vi "FT_Read_FT232H_EEPROM.vi"(0 "Handle":u32) -> (1 "FT_Status":u32(ring) items=["FT_OK", "FT_INVALID_HANDLE", "FT_DEVICE_NOT_FOUND", "FT_DEVICE_NOT_OPENED", "FT_IO_ERROR", "FT_INSUFFICIENT_RESOURCES", "FT_INVALID_PARAMETER", "FT_INVALID_BAUD_RATE", "FT_DEVICE_NOT_OPENED_FOR_ERASE", "FT_DEVICE_NOT_OPENED_FOR_WRITE", "FT_FAILED_TO_WRITE_DEVICE", "FT_EEPROM_READ_FAILED", "FT_EEPROM_WRITE_FAILED", "FT_EEPROM_ERASE_FAILED", "FT_EEPROM_NOT_PRESENT", "FT_EEPROM_NOT_PROGRAMMED", "FT_INVALID_ARGS", "FT_NOT_SUPPORTED", "FT_OTHER_ERROR"], 2 "FT232H EEPROM Contents":T1={"Vendor ID"=0, "Product ID"=0, "Manufacturer"="", "Manufacturer ID"="", "Description"="", "Serial Number"="", "Max Power (mA)"=0, "PnP"=0, "Self Powered"=0, "Remote Wake-Up"=0, "Pull Down Enable"=0, "Serial Number Enable"=0, "AC Slow Slew"=0, "AC Schmitt Input"=0, "AC Drive Current"=4, "AD Slow Slew"=0, "AD Schmitt Input"=0, "AD Drive Current"=4, "CBus0"=0, "CBus1"=0, "CBus2"=0, "CBus3"=0, "CBus4"=0, "CBus5"=0, "CBus6"=0, "CBus7"=0, "CBus8"=0, "CBus9"=0, "Is 245 FIFO"=0, "Is CPU FIFO"=0, "Is Fast Serial"=0, "Is FT1248"=0, "FT1248 Clock Polarity"=0, "FT1248 Bit Order"=0, "FT1248 Flow Control"=0, "Is VCP"=0, "Power Save"=0} {"Power Save" items=["Disabled", "Enabled"]; "Is VCP" items=["D2XX", "VCP"]; "FT1248 Flow Control" items=["Disabled", "Enabled"]; "FT1248 Bit Order" items=["MSB", "LSB"]; "FT1248 Clock Polarity" items=["Idle Low", "Idle High"]; "Is FT1248" items=["Disabled", "Enabled"]; "Is Fast Serial" items=["Disabled", "Enabled"]; "Is CPU FIFO" items=["Disabled", "Enabled"]; "Is 245 FIFO" items=["UART", "FIFO"]; "CBus9" items=["TRISTATE", "RXLED#", "TXLED#", "TX & RXLED#", "PWREN#", "SLEEP#", "DRIVE 0", "DRIVE 1", "IO Mode", "TXDEN#", "30MHz Clock", "15MHz Clock", "7.5MHz Clock"]; "CBus8" items=["TRISTATE", "RXLED#", "TXLED#", "TX & RXLED#", "PWREN#", "SLEEP#", "DRIVE 0", "DRIVE 1", "IO Mode", "TXDEN#", "30MHz Clock", "15MHz Clock", "7.5MHz Clock"]; "CBus7" items=["TRISTATE", "RXLED#", "TXLED#", "TX & RXLED#", "PWREN#", "SLEEP#", "DRIVE 0", "DRIVE 1", "IO Mode", "TXDEN#", "30MHz Clock", "15MHz Clock", "7.5MHz Clock"]; "CBus6" items=["TRISTATE", "RXLED#", "TXLED#", "TX & RXLED#", "PWREN#", "SLEEP#", "DRIVE 0", "DRIVE 1", "IO Mode", "TXDEN#", "30MHz Clock", "15MHz Clock", "7.5MHz Clock"]; "CBus5" items=["TRISTATE", "RXLED#", "TXLED#", "TX & RXLED#", "PWREN#", "SLEEP#", "DRIVE 0", "DRIVE 1", "IO Mode", "TXDEN#", "30MHz Clock", "15MHz Clock", "7.5MHz Clock"]; "CBus4" items=["TRISTATE", "RXLED#", "TXLED#", "TX & RXLED#", "PWREN#", "SLEEP#", "DRIVE 0", "DRIVE 1", "IO Mode", "TXDEN#", "30MHz Clock", "15MHz Clock", "7.5MHz Clock"]; "CBus3" items=["TRISTATE", "RXLED#", "TXLED#", "TX & RXLED#", "PWREN#", "SLEEP#", "DRIVE 0", "DRIVE 1", "IO Mode", "TXDEN#", "30MHz Clock", "15MHz Clock", "7.5MHz Clock"]; "CBus2" items=["TRISTATE", "RXLED#", "TXLED#", "TX & RXLED#", "PWREN#", "SLEEP#", "DRIVE 0", "DRIVE 1", "IO Mode", "TXDEN#", "30MHz Clock", "15MHz Clock", "7.5MHz Clock"]; "CBus1" items=["TRISTATE", "RXLED#", "TXLED#", "TX & RXLED#", "PWREN#", "SLEEP#", "DRIVE 0", "DRIVE 1", "IO Mode", "TXDEN#", "30MHz Clock", "15MHz Clock", "7.5MHz Clock"]; "CBus0" items=["TRISTATE", "RXLED#", "TXLED#", "TX & RXLED#", "PWREN#", "SLEEP#", "DRIVE 0", "DRIVE 1", "IO Mode", "TXDEN#", "30MHz Clock", "15MHz Clock", "7.5MHz Clock"]; "AD Drive Current" items=["4mA"=4, "8mA"=8, "12mA"=12, "16mA"=16]; "AD Schmitt Input" items=["Disabled", "Enabled"]; "AD Slow Slew" items=["Disabled", "Enabled"]; "AC Drive Current" items=["4mA"=4, "8mA"=8, "12mA"=12, "16mA"=16]; "AC Schmitt Input" items=["Disabled", "Enabled"]; "AC Slow Slew" items=["Disabled", "Enabled"]; "Serial Number Enable" items=["Disabled", "Enabled"]; "Pull Down Enable" items=["Disabled", "Enabled"]; "Remote Wake-Up" items=["Disabled", "Enabled"]; "Self Powered" items=["Bus Powered", "Self Powered"]; "PnP" items=["Disabled", "Enabled"]; "Product ID" format="%x"; "Vendor ID" format="%x"})   [LabVIEW 2020]
uses:
  GEA3 DLL Source/ftd2xx.dll
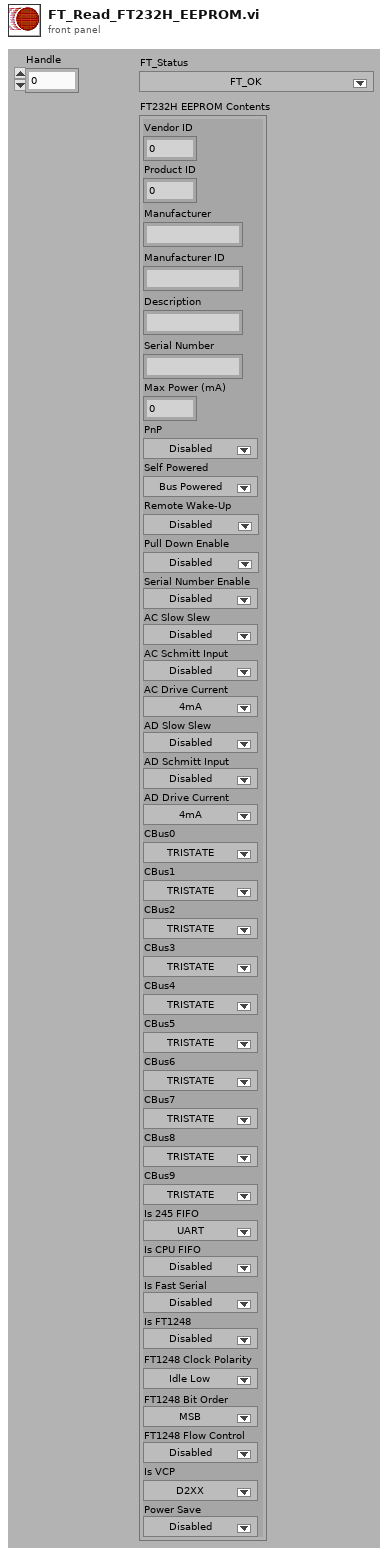
[diagram p1: front panel]
types:
  T1 = cluster{"Vendor ID":u16, "Product ID":u16, "Manufacturer":string, "Manufacturer ID":string, "Description":string, "Serial Number":string, "Max Power (mA)":u16, "PnP":u16, "Self Powered":u16, "Remote Wake-Up":u16, "Pull Down Enable":u8, "Serial Number Enable":u8, "AC Slow Slew":u8, "AC Schmitt Input":u8, "AC Drive Current":u8, "AD Slow Slew":u8, "AD Schmitt Input":u8, "AD Drive Current":u8, "CBus0":u8, "CBus1":u8, "CBus2":u8, "CBus3":u8, "CBus4":u8, "CBus5":u8, "CBus6":u8, "CBus7":u8, "CBus8":u8, "CBus9":u8, "Is 245 FIFO":u8, "Is CPU FIFO":u8, "Is Fast Serial":u8, "Is FT1248":u8, "FT1248 Clock Polarity":u8, "FT1248 Bit Order":u8, "FT1248 Flow Control":u8, "Is VCP":u8, "Power Save":u8}
  T2 = cluster{"Signature 1":u32, "Signature 2":u32, "Version":u32, "Vendor ID":u16, "Product ID":u16, "Manufacturer":u32, "Manufacturer ID":u32, "Description":u32, "Serial Number":u32, "Max Power (mA)":u16, "PnP":u16, "Self Powered":u16, "Remote Wake-Up":u16, "Rev4":u8, "Iso In":u8, "Iso Out":u8, "Pull Down Enable":u8, "Serial Number Enable":u8, "USB Version Enable":u8, "USB Version":u16, "Rev5":u8, "Iso In A":u8, "Iso In B":u8, "Iso Out A":u8, "Iso Out B":u8, "Pull Down Enable 5":u8, "Serial Number Enable 5":u8, "USB Version Enable 5":u8, "USB Version 5":u16, "A Is High Current":u8, "B Is High Current":u8, "A Is 245 FIFO":u8, "A Is CPU FIFO":u8, "A Is Fast Serial":u8, "A Is VCP":u8, "B Is 245 FIFO":u8, "B Is CPU FIFO":u8, "B Is Fast Serial":u8, "B Is VCP":u8, "Use Ext Osc":u8, "High Drive IOs":u8, "Endpoint Size":u8, "Pull Down Enable R":u8, "Serial Number Enable R":u8, "Invert TXD":u8, "Invert RXD":u8, "Invert RTS":u8, "Invert CTS":u8, "Invert DTR":u8, "Invert DSR":u8, "Invert DCD":u8, "Invert RI":u8, "CBus0":u8, "CBus1":u8, "CBus2":u8, "CBus3":u8, "CBus4":u8, "R Is VCP":u8, "Pull Down Enable 7":u8, "Serial Number Enable 7":u8, "AL Slow Slew":u8, "AL Schmitt Input":u8, "AL Drive Current":u8, "AH Slow Slew":u8, "AH Schmitt Input":u8, "AH Drive Current":u8, "BL Slow Slew":u8, "BL Schmitt Input":u8, "BL Drive Current":u8, "BH Slow Slew":u8, "BH Schmitt Input":u8, "BH Drive Current":u8, "A Is 245 FIFO 7":u8, "A Is CPU FIFO 7":u8, "A Is Fast Serial 7":u8, "A Is VCP 7":u8, "B Is 245 FIFO 7":u8, "B Is CPU FIFO 7":u8, "B Is Fast Serial 7":u8, "B Is VCP 7":u8, "PowerSaveEnable":u8, "Pull Down Enable 8":u8, "Serial Number Enable 8":u8, "A Slow Slew":u8, "A Schmitt Input":u8, "A Drive Current":u8, "B Slow Slew":u8, "B Schmitt Input":u8, "B Drive Current":u8, "C Slow Slew":u8, "C Schmitt Input":u8, "C Drive Current":u8, "D Slow Slew":u8, "D Schmitt Input":u8, "D Drive Current":u8, "A RI Is TXDEN":u8, "B RI Is TXDEN":u8, "C RI Is TXDEN":u8, "D RI Is TXDEN":u8, "A Is VCP 8":u8, "B Is VCP 8":u8, "C Is VCP 8":u8, "D Is VCP 8":u8, "Pull Down Enable H":u8, "Serial Number Enable H":u8, "AC Slow Slew H":u8, "AC Schmitt Input H":u8, "AC Drive Current H":u8, "AD Slow Slew H":u8, "AD Schmitt Input H":u8, "AD Drive Current H":u8, "CBus0 H":u8, "CBus1 H":u8, "CBus2 H":u8, "CBus3 H":u8, "CBus4 H":u8, "CBus5 H":u8, "CBus6 H":u8, "CBus7 H":u8, "CBus8 H":u8, "CBus9 H":u8, "Is 245 FIFO H":u8, "Is CPU FIFO H":u8, "Is Fast Serial H":u8, "Is FT1248 H":u8, "FT1248 Clock Polarity H":u8, "FT1248 LSB H":u8, "FT1248 Flow Control H":u8, "Is VCP H":u8, "Power Save Enable H":u8}
  T3 = cluster{"Vendor ID":u16, "Product ID":u16, "Manufacturer":string, "Manufacturer ID":string, "Description":string, "Serial Number":string, "Max Power (mA)":u16, "PnP":u16, "Self Powered":u16, "Remote Wake-Up":u16, "Pull Down Enable H":u8, "Serial Number Enable H":u8, "AC Slow Slew H":u8, "AC Schmitt Input H":u8, "AC Drive Current H":u8, "AD Slow Slew H":u8, "AD Schmitt Input H":u8, "AD Drive Current H":u8, "CBus0 H":u8, "CBus1 H":u8, "CBus2 H":u8, "CBus3 H":u8, "CBus4 H":u8, "CBus5 H":u8, "CBus6 H":u8, "CBus7 H":u8, "CBus8 H":u8, "CBus9 H":u8, "Is 245 FIFO H":u8, "Is CPU FIFO H":u8, "Is Fast Serial H":u8, "Is FT1248 H":u8, "FT1248 Clock Polarity H":u8, "FT1248 LSB H":u8, "FT1248 Flow Control H":u8, "Is VCP H":u8, "Power Save Enable H":u8}
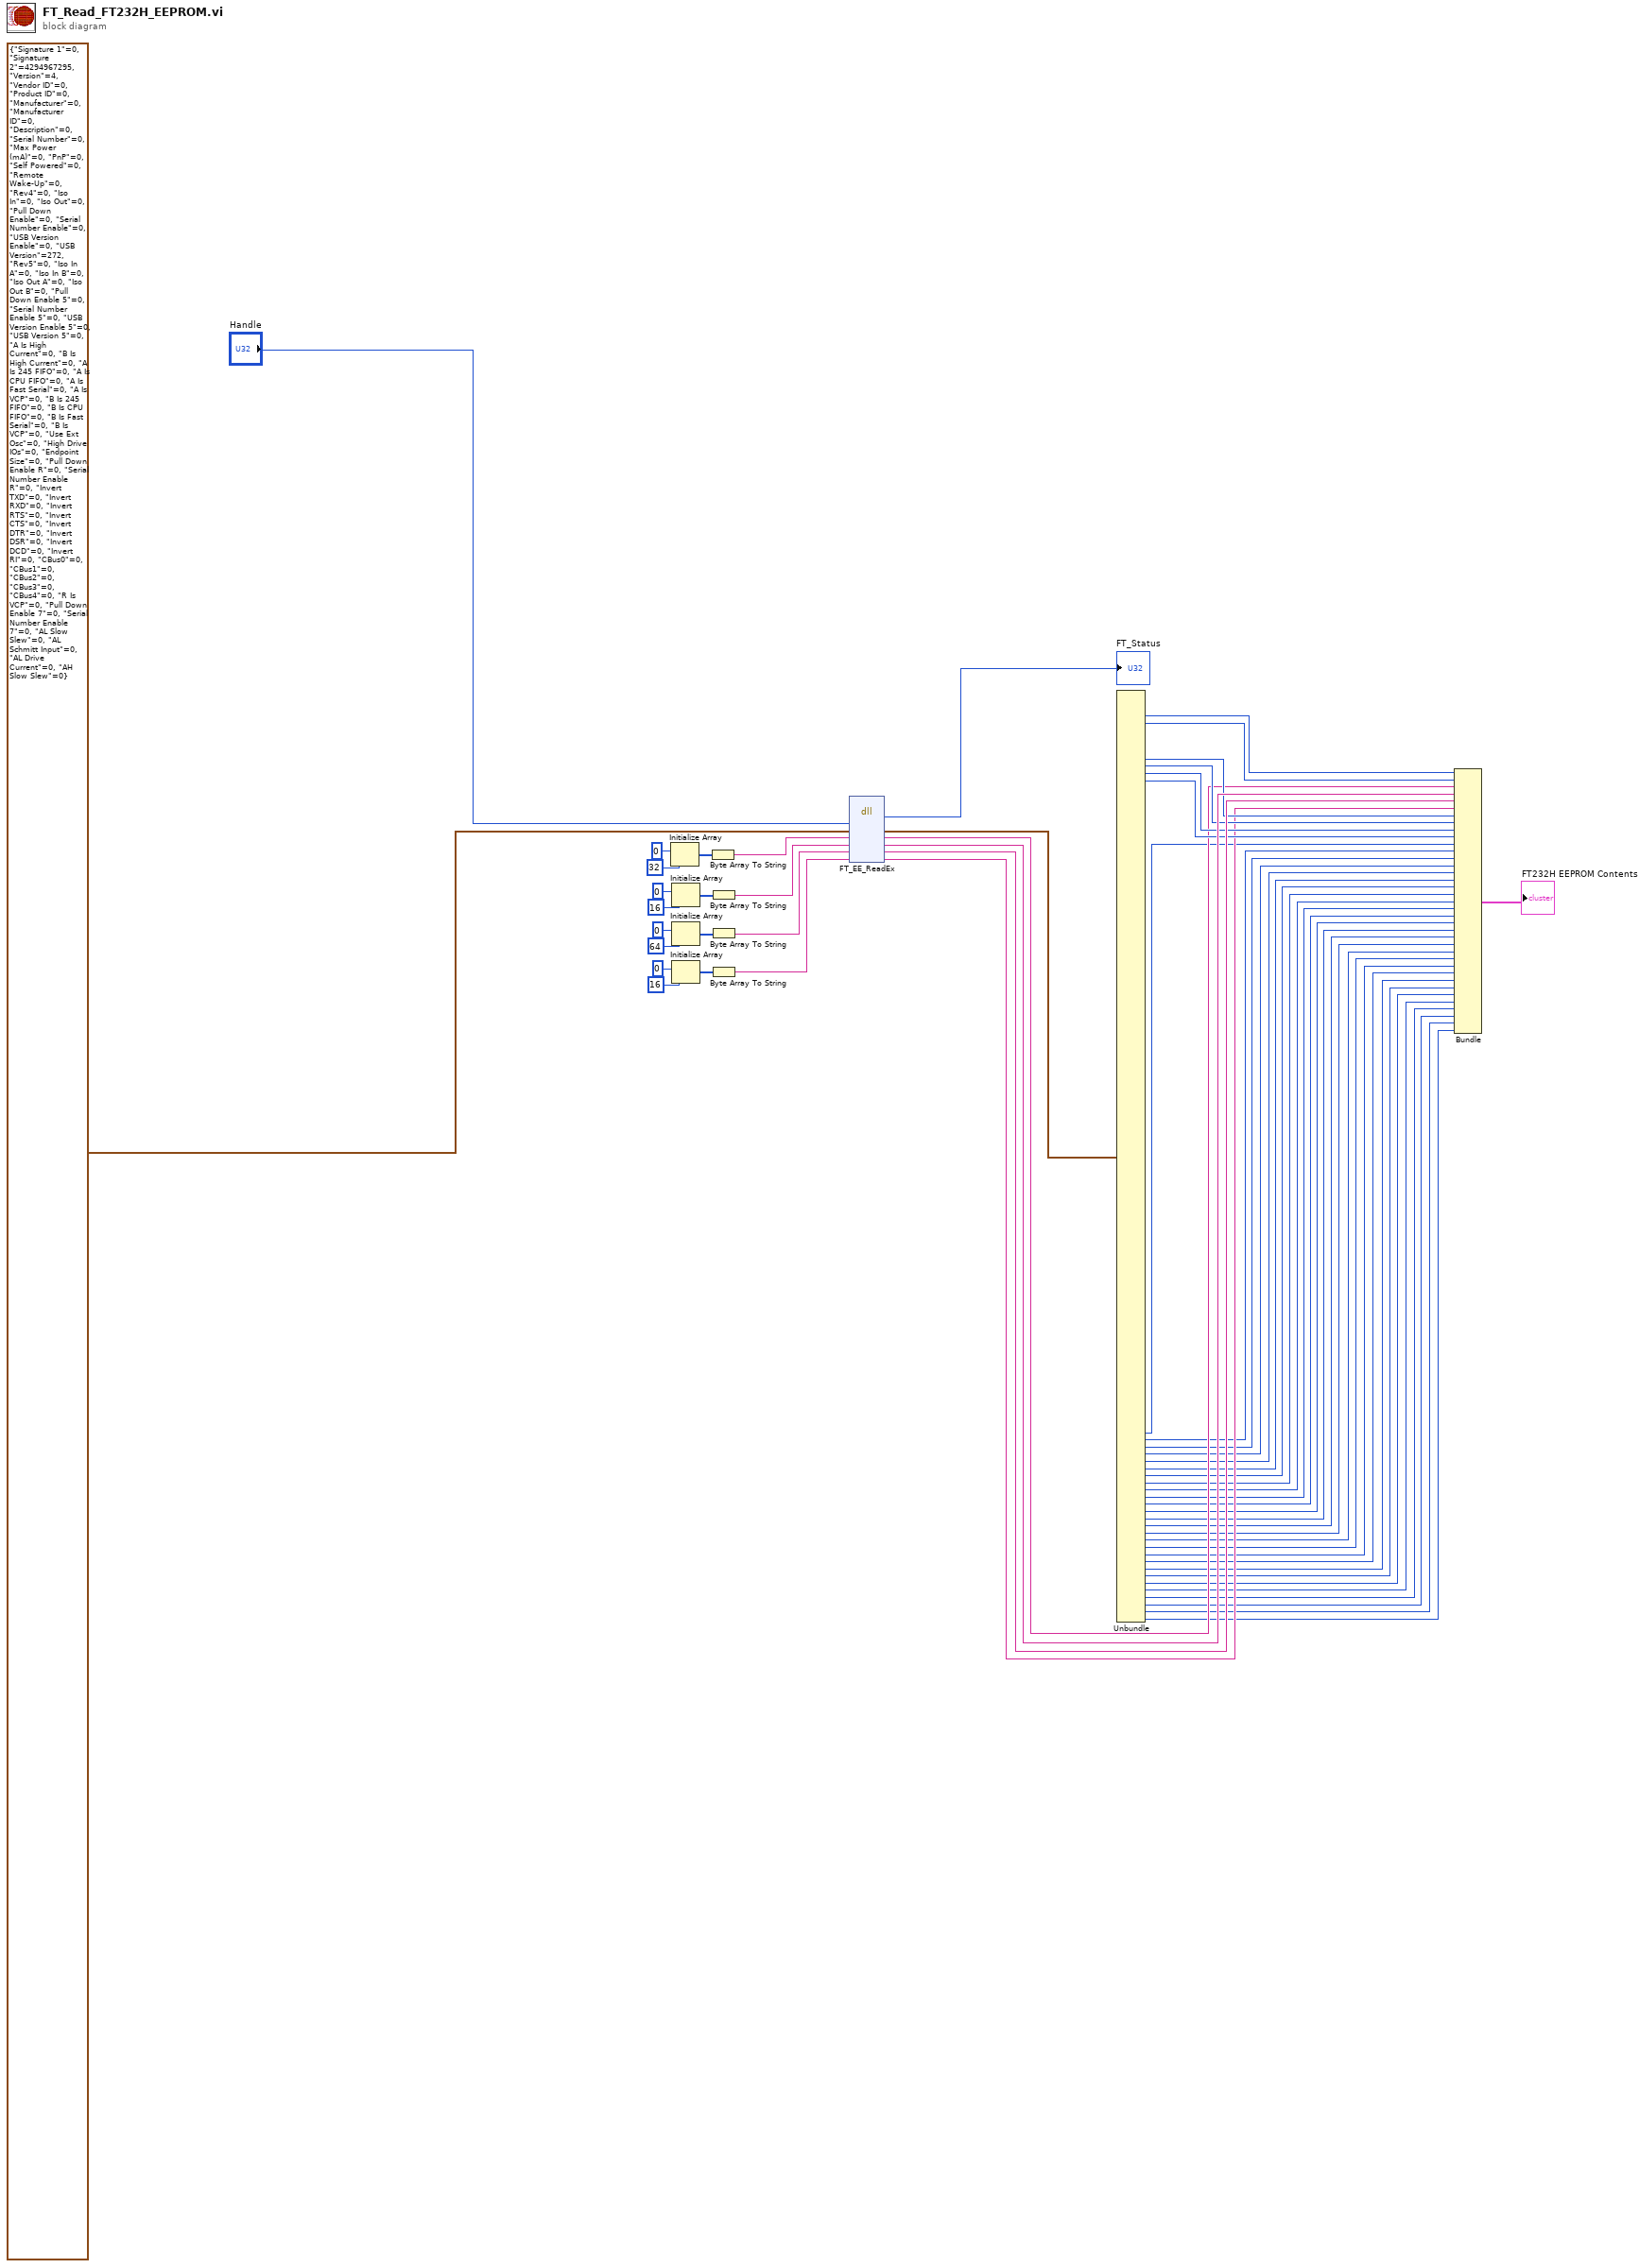
[diagram p0: block diagram]
diagram:
  n1 = Initialize Array(u8 0, 32 ("dimension size")) -> (w44:u8[])
  n2 = Initialize Array(u8 0, 16 ("dimension size")) -> (w42:u8[])
  n3 = Initialize Array(u8 0, 64 ("dimension size")) -> (w40:u8[])
  n4 = Initialize Array(u8 0, 16 ("dimension size")) -> (w38:u8[])
  n5 = Byte Array To String(unsigned byte array=w44) -> (string=w33:string)
  n6 = Byte Array To String(unsigned byte array=w42) -> (string=w32:string)
  n7 = Byte Array To String(unsigned byte array=w40) -> (string=w31:string)
  n8 = Byte Array To String(unsigned byte array=w38) -> (string=w30:string)
  n9 = dll-call lib="C:/TechnologyLab/NI-2010/Drivers/GEA3 Toolkit/GEA3 DLL Source/FTD2XX.dll" fn="FT_EE_ReadEx"("Handle"="Handle", "FT232-FT245 EEPROM Contents 4"=T2 {"Signature 1"=0, "Signature 2"=4294967295, "Version"=4, "Vendor ID"=0, "Product ID"=0, "Manufacturer"=0, "Manufacturer ID"=0, "Description"=0, "Serial Number"=0, "Max Power (mA)"=0, "PnP"=0, "Self Powered"=0, "Remote Wake-Up"=0, "Rev4"=0, "Iso In"=0, "Iso Out"=0, "Pull Down Enable"=0, "Serial Number Enable"=0, "USB Version Enable"=0, "USB Version"=272, "Rev5"=0, "Iso In A"=0, "Iso In B"=0, "Iso Out A"=0, "Iso Out B"=0, "Pull Down Enable 5"=0, "Serial Number Enable 5"=0, "USB Version Enable 5"=0, "USB Version 5"=0, "A Is High Current"=0, "B Is High Current"=0, "A Is 245 FIFO"=0, "A Is CPU FIFO"=0, "A Is Fast Serial"=0, "A Is VCP"=0, "B Is 245 FIFO"=0, "B Is CPU FIFO"=0, "B Is Fast Serial"=0, "B Is VCP"=0, "Use Ext Osc"=0, "High Drive IOs"=0, "Endpoint Size"=0, "Pull Down Enable R"=0, "Serial Number Enable R"=0, "Invert TXD"=0, "Invert RXD"=0, "Invert RTS"=0, "Invert CTS"=0, "Invert DTR"=0, "Invert DSR"=0, "Invert DCD"=0, "Invert RI"=0, "CBus0"=0, "CBus1"=0, "CBus2"=0, "CBus3"=0, "CBus4"=0, "R Is VCP"=0, "Pull Down Enable 7"=0, "Serial Number Enable 7"=0, "AL Slow Slew"=0, "AL Schmitt Input"=0, "AL Drive Current"=0, "AH Slow Slew"=0, "AH Schmitt Input"=0, "AH Drive Current"=0, "BL Slow Slew"=0, "BL Schmitt Input"=0, "BL Drive Current"=0, "BH Slow Slew"=0, "BH Schmitt Input"=0, "BH Drive Current"=0, "A Is 245 FIFO 7"=0, "A Is CPU FIFO 7"=0, "A Is Fast Serial 7"=0, "A Is VCP 7"=0, "B Is 245 FIFO 7"=0, "B Is CPU FIFO 7"=0, "B Is Fast Serial 7"=0, "B Is VCP 7"=0, "PowerSaveEnable"=0, "Pull Down Enable 8"=0, "Serial Number Enable 8"=0, "A Slow Slew"=0, "A Schmitt Input"=0, "A Drive Current"=0, "B Slow Slew"=0, "B Schmitt Input"=0, "B Drive Current"=0, "C Slow Slew"=0, "C Schmitt Input"=0, "C Drive Current"=0, "D Slow Slew"=0, "D Schmitt Input"=0, "D Drive Current"=0, "A RI Is TXDEN"=0, "B RI Is TXDEN"=0, "C RI Is TXDEN"=0, "D RI Is TXDEN"=0, "A Is VCP 8"=0, "B Is VCP 8"=0, "C Is VCP 8"=0, "D Is VCP 8"=0, "Pull Down Enable H"=0, "Serial Number Enable H"=0, "AC Slow Slew H"=0, "AC Schmitt Input H"=0, "AC Drive Current H"=0, "AD Slow Slew H"=0, "AD Schmitt Input H"=0, "AD Drive Current H"=0, "CBus0 H"=0, "CBus1 H"=0, "CBus2 H"=0, "CBus3 H"=0, "CBus4 H"=0, "CBus5 H"=0, "CBus6 H"=0, "CBus7 H"=0, "CBus8 H"=0, "CBus9 H"=0, "Is 245 FIFO H"=0, "Is CPU FIFO H"=0, "Is Fast Serial H"=0, "Is FT1248 H"=0, "FT1248 Clock Polarity H"=0, "FT1248 LSB H"=0, "FT1248 Flow Control H"=0, "Is VCP H"=0, "Power Save Enable H"=0}, "Manufacturer"=w33, "Manufacturer ID"=w32, "Description"=w31, "Serial Number"=w30) -> ("FT_Status"=→"FT_Status":u32, "FT232-FT245 EEPROM Contents 4"=w56:T2, "Manufacturer"=w47:string, "Manufacturer ID"=w53:string, "Description"=w52:string, "Serial Number"=w46:string)  [unwired: 4 in, 2 out]
  n10 = Unbundle(w56) -> ("Vendor ID"=w55:u16, "Product ID"=w54:u16, "Max Power (mA)"=w51:u16, "PnP"=w50:u16, "Self Powered"=w49:u16, "Remote Wake-Up"=w48:u16, "Pull Down Enable H"=w28:u8, "Serial Number Enable H"=w27:u8, "AC Slow Slew H"=w26:u8, "AC Schmitt Input H"=w25:u8, "AC Drive Current H"=w24:u8, "AD Slow Slew H"=w23:u8, "AD Schmitt Input H"=w22:u8, "AD Drive Current H"=w21:u8, "CBus0 H"=w20:u8, "CBus1 H"=w19:u8, "CBus2 H"=w18:u8, "CBus3 H"=w17:u8, "CBus4 H"=w16:u8, "CBus5 H"=w15:u8, "CBus6 H"=w14:u8, "CBus7 H"=w13:u8, "CBus8 H"=w12:u8, "CBus9 H"=w11:u8, "Is 245 FIFO H"=w10:u8, "Is CPU FIFO H"=w9:u8, "Is Fast Serial H"=w8:u8, "Is FT1248 H"=w5:u8, "FT1248 Clock Polarity H"=w4:u8, "FT1248 LSB H"=w3:u8, "FT1248 Flow Control H"=w2:u8, "Is VCP H"=w1:u8, "Power Save Enable H"=w6:u8)  [unwired: 97 out]
  n11 = Bundle("Vendor ID"=w55, "Product ID"=w54, "Manufacturer"=w47, "Manufacturer ID"=w53, "Description"=w52, "Serial Number"=w46, "Max Power (mA)"=w51, "PnP"=w50, "Self Powered"=w49, "Remote Wake-Up"=w48, "Pull Down Enable H"=w28, "Serial Number Enable H"=w27, "AC Slow Slew H"=w26, "AC Schmitt Input H"=w25, "AC Drive Current H"=w24, "AD Slow Slew H"=w23, "AD Schmitt Input H"=w22, "AD Drive Current H"=w21, "CBus0 H"=w20, "CBus1 H"=w19, "CBus2 H"=w18, "CBus3 H"=w17, "CBus4 H"=w16, "CBus5 H"=w15, "CBus6 H"=w14, "CBus7 H"=w13, "CBus8 H"=w12, "CBus9 H"=w11, "Is 245 FIFO H"=w10, "Is CPU FIFO H"=w9, "Is Fast Serial H"=w8, "Is FT1248 H"=w5, "FT1248 Clock Polarity H"=w4, "FT1248 LSB H"=w3, "FT1248 Flow Control H"=w2, "Is VCP H"=w1, "Power Save Enable H"=w6) -> (→"FT232H EEPROM Contents":T3)  [unwired: 1 in]
